vi "AdquisicioDadesAkan.vi"(8 "Stop":refnum<vi>, 10 "user event":refnum<user-event>) -> ()   [LabVIEW 2017]
uses:
  <vilib>/DAQmx/read.llb/DAQmx Read (Analog 2D DBL NChan NSamp).vi
  <vilib>/DAQmx/miscellaneous.llb/DAQmx Fill In Error Info.vi
  <resource>/objmgr/daqmx.rc
panel:
  out "appended array":dbl[](array[numeric]) format="%#_8g"
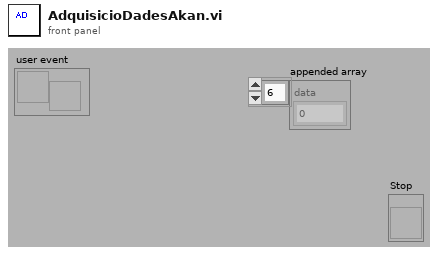
[diagram p1: front panel]
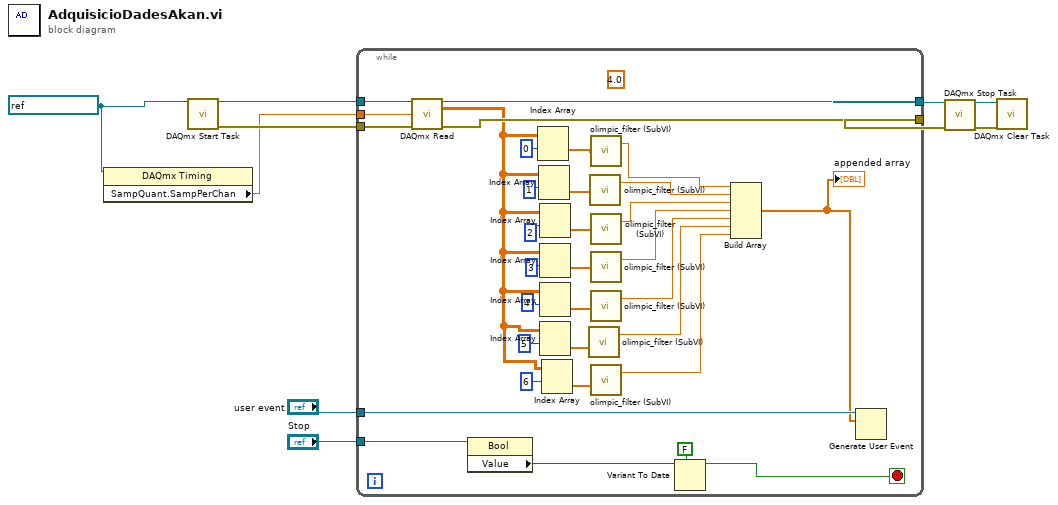
[diagram p0: block diagram]
diagram:
  w2 = refnum<k21> "AkanCables" ("task/channels in")
  n1 = property class="DAQmx Timing"(reference=w2) -> ("SampQuant.SampPerChan"=w1:dbl)  [unwired: 1 in, 2 out]
  n2 = call <vilib>:"DAQmx Start Task.vi"("task/channels in"=w2) -> ("task out"=w9:refnum<k21>, "error out"=w8:errorcluster)  [unwired: 13 in]
  n3 = while {
    tunnel: w9 -> [w35]
    tunnel: [w36] -> w10
    tunnel: w8 -> [w43]
    tunnel: "Stop" -> [w42]
    tunnel: [w39] -> w6
    tunnel: "user event" -> [w37]
    tunnel: w1 -> [w34]
    stop <- w38 stop-if-true
    (unwired) 4.0 ("Lower Cut-Off")
    n4 = call-poly <vilib>:"DAQmx Read.vi"("task/channels in"=w35, "number of samples per channel"=w34, "error in"=w43) -> ("task out"=w36:refnum<k21>, "data"=w20:dbl[][], "error out"=w39:errorcluster)  [unwired: 10 in]
    n5 = property class="Bool"(reference=w42) -> ("Value"=w41:variant)  [unwired: 1 in, 2 out]
    n6 = Index Array(array=w20, index (row)=0) -> (element=w12:dbl[])  [unwired: 1 in]
    n7 = Index Array(array=w20, index (row)=1) -> (element=w27:dbl[])  [unwired: 1 in]
    n8 = Index Array(array=w20, index (row)=2) -> (element=w26:dbl[])  [unwired: 1 in]
    n9 = Index Array(array=w20, index (row)=3) -> (element=w29:dbl[])  [unwired: 1 in]
    n10 = Index Array(array=w20, index (row)=4) -> (element=w25:dbl[])  [unwired: 1 in]
    n11 = Index Array(array=w20, index (row)=5) -> (element=w23:dbl[])  [unwired: 1 in]
    n12 = Index Array(array=w20, index (row)=6) -> (element=w21:dbl[])  [unwired: 1 in]
    n13 = call "olimpic_filter (SubVI).vi"("array"=w23) -> ("olimpic_filter"=w15:dbl)  [unwired: 1 out]
    n14 = call "olimpic_filter (SubVI).vi"("array"=w27) -> ("olimpic_filter"=w19:dbl)  [unwired: 1 out]
    n15 = call "olimpic_filter (SubVI).vi"("array"=w12) -> ("olimpic_filter"=w11:dbl)  [unwired: 1 out]
    n16 = call "olimpic_filter (SubVI).vi"("array"=w26) -> ("olimpic_filter"=w18:dbl)  [unwired: 1 out]
    n17 = call "olimpic_filter (SubVI).vi"("array"=w29) -> ("olimpic_filter"=w17:dbl)  [unwired: 1 out]
    n18 = call "olimpic_filter (SubVI).vi"("array"=w25) -> ("olimpic_filter"=w16:dbl)  [unwired: 1 out]
    n19 = call "olimpic_filter (SubVI).vi"("array"=w21) -> ("olimpic_filter"=w14:dbl)  [unwired: 1 out]
    n20 = Variant To Data(type=FALSE, Variant=w41) -> (data=w38:bool)  [unwired: 1 in, 1 out]
    n21 = Build Array(w11, w19, w18, w17, w16, w15, w14) -> (w13:dbl[])
    "appended array" <- w13
    n22 = Generate User Event(user event=w37, event data cluster=w13) -> ()  [unwired: 2 in, 2 out]
  }
  n23 = call <vilib>:"DAQmx Stop Task.vi"("task/channels in"=w10, "error in"=w6) -> ("task out"=w4:refnum<k21>, "error out"=w3:errorcluster)  [unwired: 12 in]
  n24 = call <vilib>:"DAQmx Clear Task.vi"("task in"=w4, "error in"=w3) -> ()  [unwired: 13 in, 1 out]
